vi "Facade.vi"(0 "Data In":T5 {"Stages"."IIR Filter"."Forward Coefficients" format="%.4f"; "Stages"."IIR Filter"."Reverse Coefficients" format="%.4f"}, 2 "Display State In":T3, 3 "Container State":T4) -> (6 "Data Out":T5 {"Stages"."IIR Filter"."Forward Coefficients" format="%.4f"; "Stages"."IIR Filter"."Reverse Coefficients" format="%.4f"}, 7 "Display State Out":T3, 8 "Action":T2)   [LabVIEW 2020, in "Advanced Filter XCtl.xctl"]
uses:
  Advanced Filter XCtl.xctl
  Filter Data.ctl
  Filter VIs/Filter-Bandwidth Units.ctl
  <vilib>/_xctls/Container State.ctl
  State.ctl
  <vilib>/_xctls/Action.ctl
  <vilib>/_xctls/XControlSupport.lvlib
panel:
  in  "BWUnits":u16(ring) caption="Filter" items=["kHz", "Octaves"]
  in  "Cascade":bool
  in  "F2":dbl caption="BW"
  in  "Type":T1(ring) caption="Filter"
  in  "F1":dbl caption="CF (kHz)"
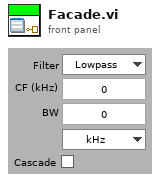
[diagram p1: front panel]
types:
  T1 = enum16{"Lowpass", "Highpass", "Bandpass", "Bandstop", "OFF"}
  T2 = typedef "XControlSupport.lvlib/Action.ctl" = cluster{"Data Changed?":bool, "State Changed?":bool, "Action Name":string}
  T3 = typedef "Advanced Filter XCtl.xctl/State.ctl" = cluster{"Show Fl/Fh?":bool}
  T4 = typedef "XControlSupport.lvlib/Container State.ctl" = cluster{"Indicator?":bool, "Run Mode?":bool, " Refnum":refnum<vi>}
  T5 = typedef "Advanced Filter XCtl.xctl/Filter Data.ctl" = cluster{"Type":enum16{"Lowpass", "Highpass", "Bandpass", "Bandstop", "OFF"}, "CF (kHz)":dbl, "BW (kHz)":dbl, "Cascade":bool, "Quadrature":bool, "Scale Factor":dbl, "Stages":cluster{"IIR Filter":cluster{"filter structure":enum32{"IIR 2nd Order", "IIR 4th Order"}, "Reverse Coefficients":dbl[], "Forward Coefficients":dbl[]}, "State":dbl[]}[], "Class":enum16{"Elliptic", "Butterworth"}, "Order":i32, "BWUnits":T6}
  T6 = typedef "Filter-Bandwidth Units.ctl" = enum16{"Linear", "Octaves", "Min-Max"}
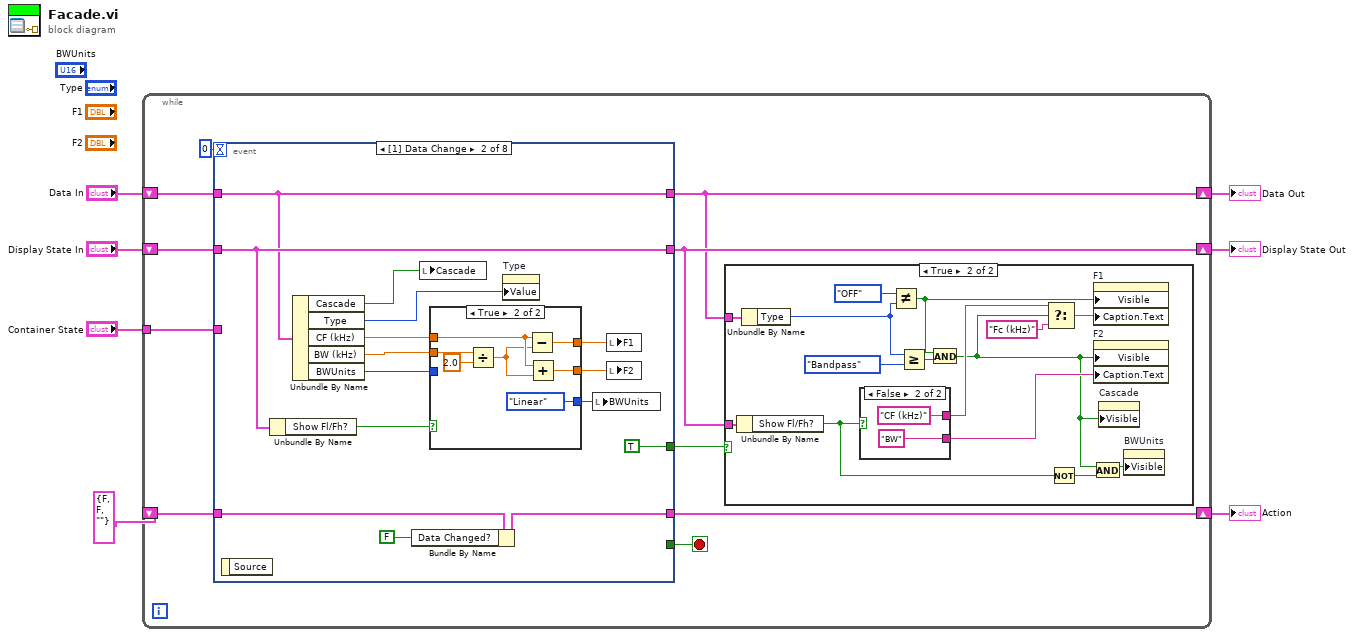
[diagram p0: block diagram]
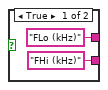
[diagram p3: hidden frame]
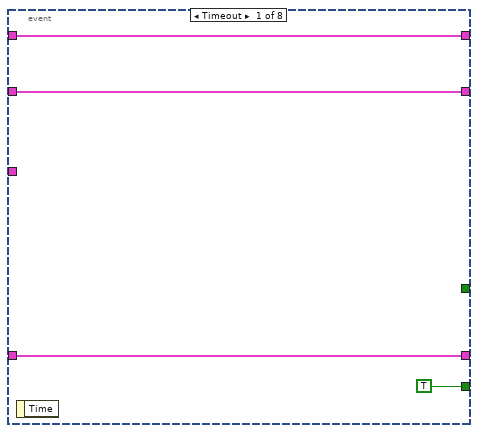
[diagram p4: hidden frame]
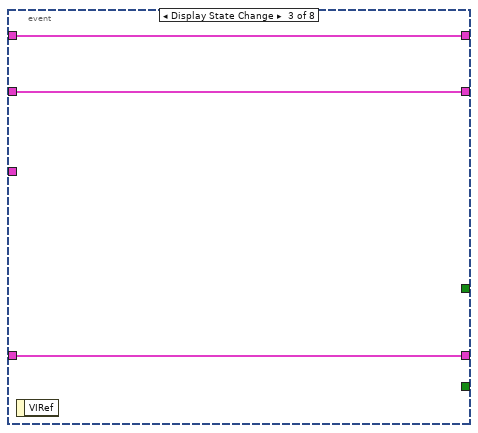
[diagram p6: hidden frame]
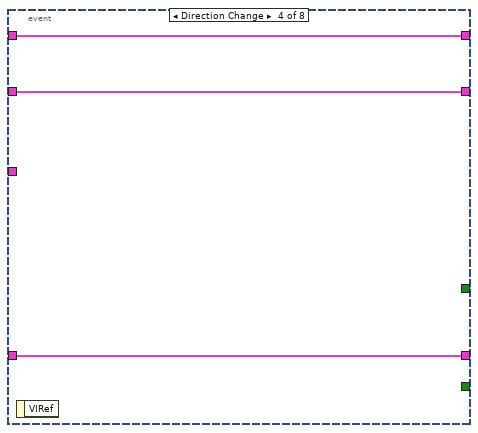
[diagram p7: hidden frame]
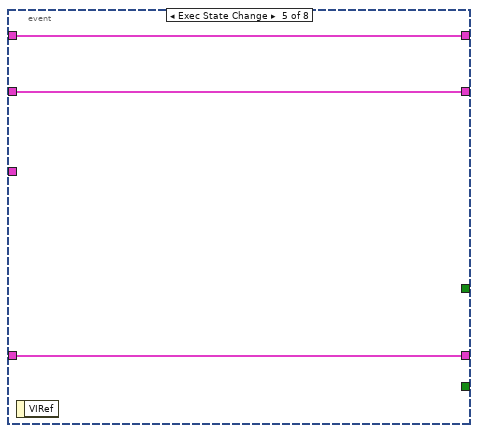
[diagram p8: hidden frame]
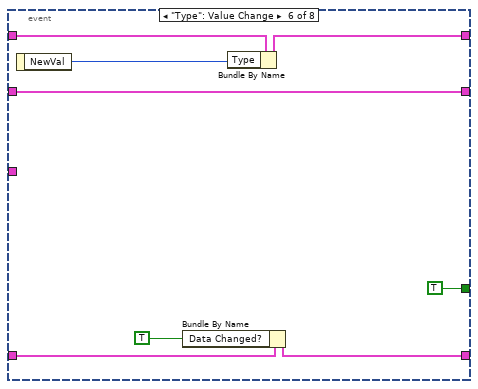
[diagram p9: hidden frame]
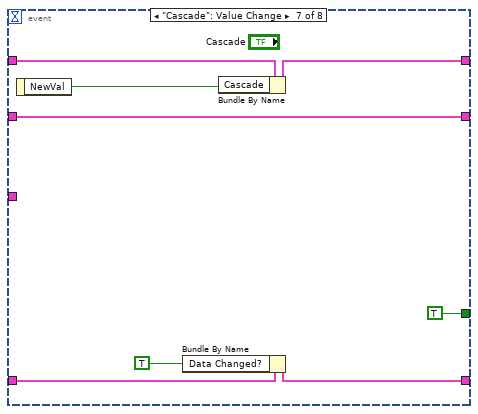
[diagram p10: hidden frame]
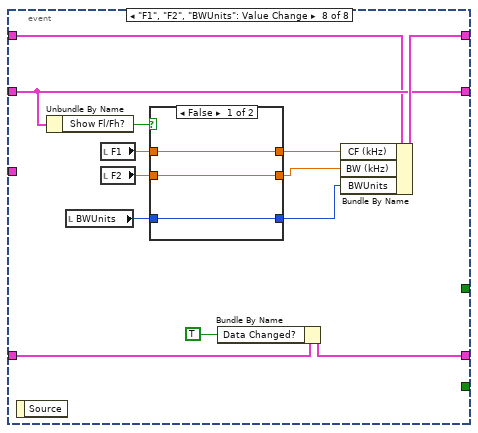
[diagram p11: hidden frame]
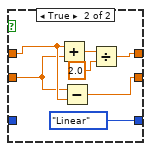
[diagram p12: hidden frame]
diagram:
  n1 = while {
    shift-right: [w10] -> w4
    shift-left: "Display State In" -> [w17]
    tunnel: "Container State" -> [w14]
    shift-right: [w9] -> w7
    shift-left: "Data In" -> [w13]
    shift-right: [w11] -> w2
    shift-left: T2 {"Data Changed?"=FALSE, "State Changed?"=FALSE, "Action Name"=""} ("Action") -> [w12]
    stop <- w16 stop-if-true
    n2 = event shown="[1] Data Change" {
      selector: _ -> [_ _ _ _ _ _ _ _]
      dyn-events: _ -> [_ _ _ _ _ _ _ _]
      timeout: 0 -> [_ _ _ _ _ _ _ _]
      tunnel: w17 -> [w38 w46 w67 w71 w74 w78 w86 w99]
      tunnel: [w38 w46 w67 w71 w74 w78 w86 w99] -> w10
      tunnel: [TRUE _ _ _ _ _ _ _] -> w16
      tunnel: w14 -> [_ _ _ _ _ _ _ _]
      tunnel: w13 -> [w37 w45 w68 w70 w73 w82 w90 w92]
      tunnel: [w37 w45 w68 w70 w73 w81 w89 w103] -> w9
      tunnel: [w39 w54 w66 w69 w72 w79 w87 w100] -> w11
      tunnel: w12 -> [w39 w55 w66 w69 w72 w80 w88 w102]
      tunnel: [_ TRUE _ _ _ TRUE TRUE _] -> w8
      event Timeout {
        n3 = event-data() -> ()  [unwired: 1 in, 1 out]
      }
      event Data Change {
        n4 = event-data() -> ()  [unwired: 1 in, 1 out]
        n5 = Unbundle By Name(w46) -> ("Show Fl/Fh?"=w52:bool)
        n6 = Unbundle By Name(w45) -> ("Cascade"=w43:bool, "Type"=w47:T1, "CF (kHz)"=w51:dbl, "BW (kHz)"=w49:dbl, "BWUnits"=w42:T6)
        n7 = Bundle By Name(cluster=w55, "Data Changed?"=FALSE) -> (w54:T2)
        n8 = local write "Cascade"(w43) -> ()
        n9 = case shown="True" w52 {
          tunnel: w51 -> [w58 w62]
          tunnel: [w58 w63] -> w50
          tunnel: [w57 w60] -> w48
          tunnel: w49 -> [w57 w65]
          tunnel: w42 -> [w56 _]
          tunnel: [w56 Filter-Bandwidth_Units."Linear" ("BWUnits")] -> w41
          frame False {
          }
          frame True {
            n10 = Divide(x=w65, y=2.0) -> (x/y=w61:dbl)
            n11 = Subtract(x=w62, y=w61) -> (x-y=w63:dbl)
            n12 = Add(x=w62, y=w61) -> (x+y=w60:dbl)
          }
        }
        n13 = property on="Type" class="Enum (strict)"("Value"=w47) -> ()  [unwired: 2 in, 2 out]
        n14 = local write "BWUnits"(w41) -> ()
        n15 = local write "F1"(w50) -> ()
        n16 = local write "F2"(w48) -> ()
      }
      event Display State Change {
        n17 = event-data() -> ()  [unwired: 1 in, 1 out]
      }
      event Direction Change {
        n18 = event-data() -> ()  [unwired: 1 in, 1 out]
      }
      event Exec State Change {
        n19 = event-data() -> ()  [unwired: 1 in, 1 out]
      }
      event "Type": Value Change {
        n20 = event-data() -> ("NewVal"=w77:T1)  [unwired: 1 in]
        n21 = Bundle By Name(cluster=w80, "Data Changed?"=TRUE) -> (w79:T2)
        n22 = Bundle By Name(cluster=w82, "Type"=w77) -> (w81:T5)
      }
      event "Cascade": Value Change {
        n23 = event-data() -> ("NewVal"=w85:bool)  [unwired: 1 in]
        n24 = Bundle By Name(cluster=w88, "Data Changed?"=TRUE) -> (w87:T2)
        n25 = Bundle By Name(cluster=w90, "Cascade"=w85) -> (w89:T5)
      }
      event "F1", "F2", "BWUnits": Value Change {
        n26 = event-data() -> ()  [unwired: 1 in, 1 out]
        n27 = Unbundle By Name(w99) -> ("Show Fl/Fh?"=w98:bool)
        n28 = local read "BWUnits"() -> (w91:u16)
        n29 = local read "F1"() -> (w97:dbl)
        n30 = local read "F2"() -> (w95:dbl)
        n31 = case shown="False" w98 {
          tunnel: w97 -> [w106 w110]
          tunnel: [w106 w112] -> w96
          tunnel: [w105 w108] -> w94
          tunnel: w95 -> [w105 w109]
          tunnel: [w104 Filter-Bandwidth_Units."Linear" ("BWUnits")] -> w93
          tunnel: w91 -> [w104 _]
          frame False {
          }
          frame True {
            n32 = Add(x=w110, y=w109) -> (x+y=w113:dbl)
            n33 = Subtract(x=w109, y=w110) -> (x-y=w108:dbl)
            n34 = Divide(x=w113, y=2.0) -> (x/y=w112:dbl)
          }
        }
        n35 = Bundle By Name(cluster=w102, "Data Changed?"=TRUE) -> (w100:T2)
        n36 = Bundle By Name(cluster=w92, "CF (kHz)"=w96, "BW (kHz)"=w94, "BWUnits"=w93) -> (w103:T5)
      }
    }
    n37 = case shown="True" w8 {
      tunnel: w10 -> [_ w23]
      tunnel: w9 -> [_ w22]
      frame False {
      }
      frame True {
        n38 = Unbundle By Name(w23) -> ("Show Fl/Fh?"=w18:bool)
        n39 = Unbundle By Name(w22) -> ("Type"=w26:T1)
        n40 = case shown="False" w18 {
          tunnel: ["FLo (kHz)" "CF (kHz)"] -> w28
          tunnel: ["FHi (kHz)" "BW"] -> w24
          frame True {
          }
          frame False {
          }
        }
        n41 = Not Equal?(x=T1."OFF" ("y"), y=w26) -> (x != y?=w30:bool)
        n42 = Greater Or Equal?(x=w26, y=T1."Bandpass") -> (x >= y?=w31:bool)
        n43 = And(x=w30, y=w31) -> (x .and. y?=w21:bool)
        n44 = Select(t=w28, s=w21, f="Fc (kHz)" ("t")) -> (s? t:f=w29:string)
        n45 = Not(x=w18) -> (.not. x?=w19:bool)
        n46 = And(x=w21, y=w19) -> (x .and. y?=w20:bool)
        n47 = property on="F1" class="DigNum (strict)"("Visible"=w30, "Caption.Text"=w29) -> ()  [unwired: 2 in, 2 out]
        n48 = property on="F2" class="DigNum (strict)"("Visible"=w21, "Caption.Text"=w24) -> ()  [unwired: 2 in, 2 out]
        n49 = property on="Cascade" class="Bool (strict)"("Visible"=w21) -> ()  [unwired: 2 in, 2 out]
        n50 = property on="BWUnits" class="Ring (strict)"("Visible"=w20) -> ()  [unwired: 2 in, 2 out]
      }
    }
  }
  "Display State Out" <- w4
  "Data Out" <- w7
  "Action" <- w2
